vi "Load Stage Limits.vi"(0 "Update Limits":bool) -> (4 "Notifier Names":string[](array[string]), 8 "Stage Limits":T1[](array[typedef]), 15 "Loaded":bool)   [LabVIEW 2020]
uses:
  Stages Limits Type Defs/Stage Limits.ctl
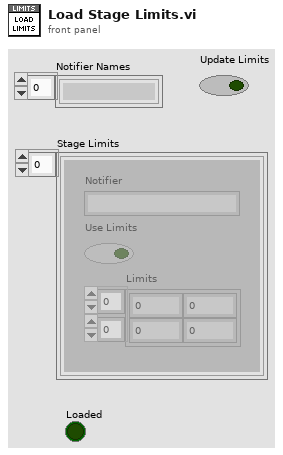
[diagram p1: front panel]
types:
  T1 = typedef "Stage Limits.ctl" = cluster{"Notifier":string, "Use Limits":bool, "Limits":dbl[][]}
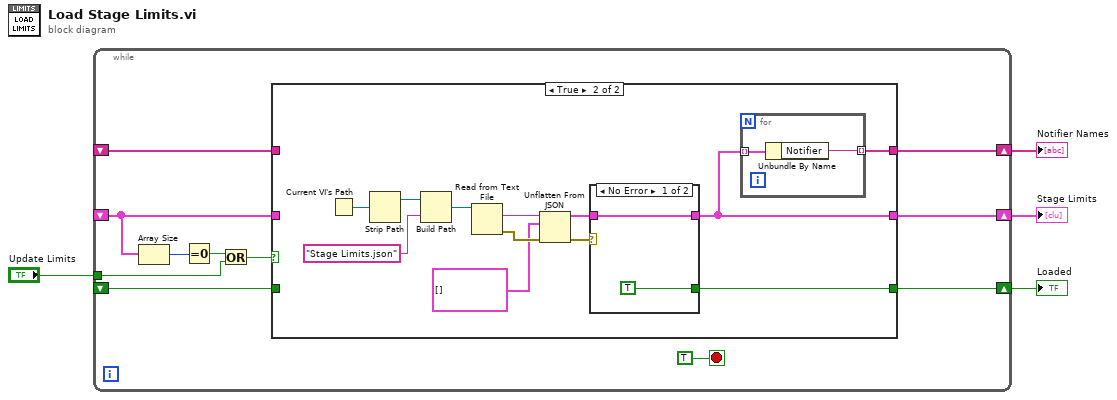
[diagram p0: block diagram]
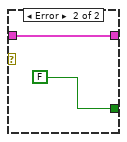
[diagram p3: hidden frame]
diagram:
  n1 = while {
    shift-right: [w14] -> w4
    shift-left: _ -> [w12]
    shift-right: [w11] -> w3
    shift-left: _ -> [w10]
    shift-right: [w9] -> w2
    shift-left: _ -> [w8]
    tunnel: "Update Limits" -> [w5]
    stop <- TRUE stop-if-true
    n2 = Array Size(array=w12) -> (size(s)=w13:i32)
    n3 = Equal To 0?(x=w13) -> (x = 0?=w7:bool)
    n4 = Or(x=w7, y=w5) -> (x .or. y?=w6:bool)
    n5 = case shown="True" w6 {
      tunnel: [w18 w24] -> w14
      tunnel: w12 -> [w18 _]
      tunnel: [w17 w25] -> w11
      tunnel: w10 -> [w17 _]
      tunnel: [w16 w23] -> w9
      tunnel: w8 -> [w16 _]
      frame False {
      }
      frame True {
        n6 = Current VI's Path() -> (path=w21:path)
        n7 = Strip Path(path=w21) -> (stripped path=w22:path)  [unwired: 1 out]
        n8 = Build Path(base path=w22, name or relative path="Stage Limits.json") -> (appended path=w19:path)
        n9 = Read from Text File(file (use dialog)=w19) -> (text=w30:string, error out=w29:errorcluster)  [unwired: 3 in, 2 out]
        n10 = Unflatten From JSON(JSON string=w30, type and defaults=T1[] [], error in (no error)=w29) -> (value=w27:T1[], error out=w28:errorcluster)  [unwired: 4 in]
        n11 = case shown="No Error" w28 {
          tunnel: w27 -> [w34 w36]
          tunnel: [w34 w36] -> w24
          tunnel: [TRUE FALSE] -> w25
          frame No Error {
          }
          frame Error {
          }
        }
        n12 = for {
          tunnel: w24 -> [w32] mode=indexing
          tunnel: [w31] -> w23 mode=indexing
          n13 = Unbundle By Name(w32) -> ("Notifier"=w31:string)
        }
      }
    }
  }
  "Stage Limits" <- w4
  "Loaded" <- w3
  "Notifier Names" <- w2
